vi "SerialTest.vi"() -> ()   [LabVIEW 2014]
doc: "This example performs a serial port write and a serial port read. The parameters set for the serial port must match the parameters of the connected instrument or device. The VISA Configure Serial Port VI sets the configuration parameters. The front panel displays the controls used to configure the basic parameters, such as baud rate, data bits, and parity. The VI passes the VISA resource name to other VIs that perform operations on that VISA resource. The VISA Write function sends a command to the serial device and the VISA Read function returns data based on the command. The VISA Close function then closes the reference to the serial device. It is important to close the reference; otherwise, further communication through that port might not be possible."
uses:
  <vilib>/Instr/_visa.llb/VISA Configure Serial Port (Instr).vi
panel:
  in  "Voltage":dbl min=0.0 max=5000.0 step=0.1 format="%.1f"
  in  "Module":i32=1 min=0 max=5 step=1
  in  "Command":T1(ring)
  out "Response 2":string
  out "Message":string
  in  "Send":bool
  in  "stop":bool
  in  "Command":string="\u000214V1=3244.0v\n"
  out "bytes read":u32
  in  "delay  (ms)":u32=200
  out "Response":string
  in  "VISA resource name":refnum<visa-resource-name>="COM8"
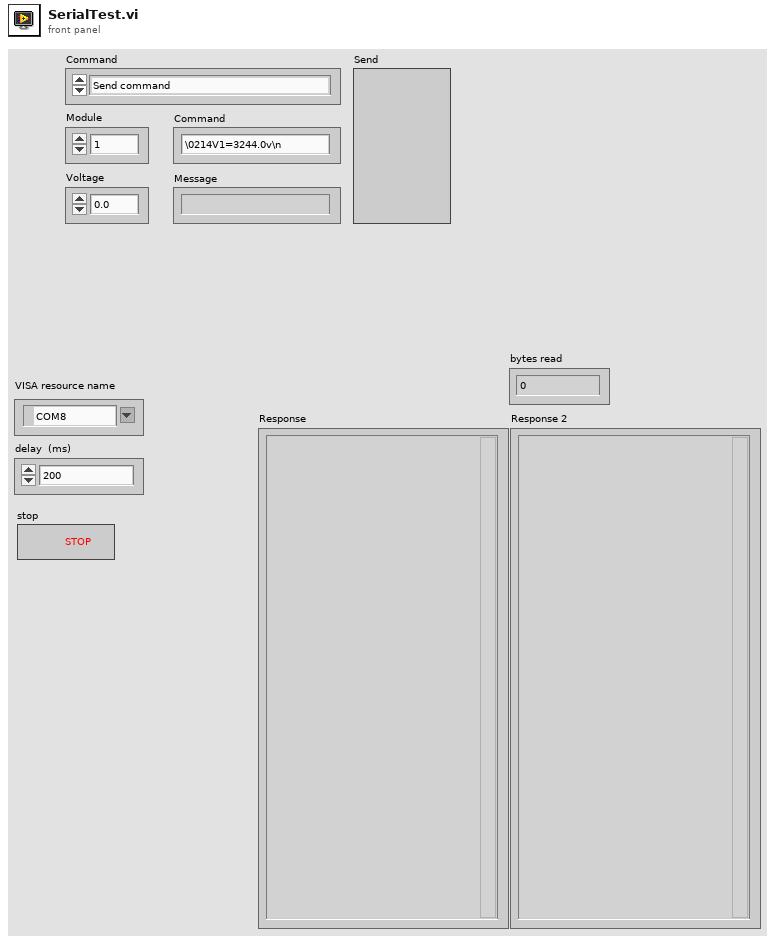
[diagram p1: front panel]
types:
  T1 = enum16{"Send command", "Reset arduino", "Get all set voltages", "Get all actual voltages", "Get all currents", "Get set voltage", "Get actual voltage", "Get current", "Set voltage"}
  T2 = cluster{"baud rate":u32, "data bits":u16, "parity":enum16{"None", "Odd", "Even", "Mark", "Space"}, "stop bits":u16, "flow control":u16}
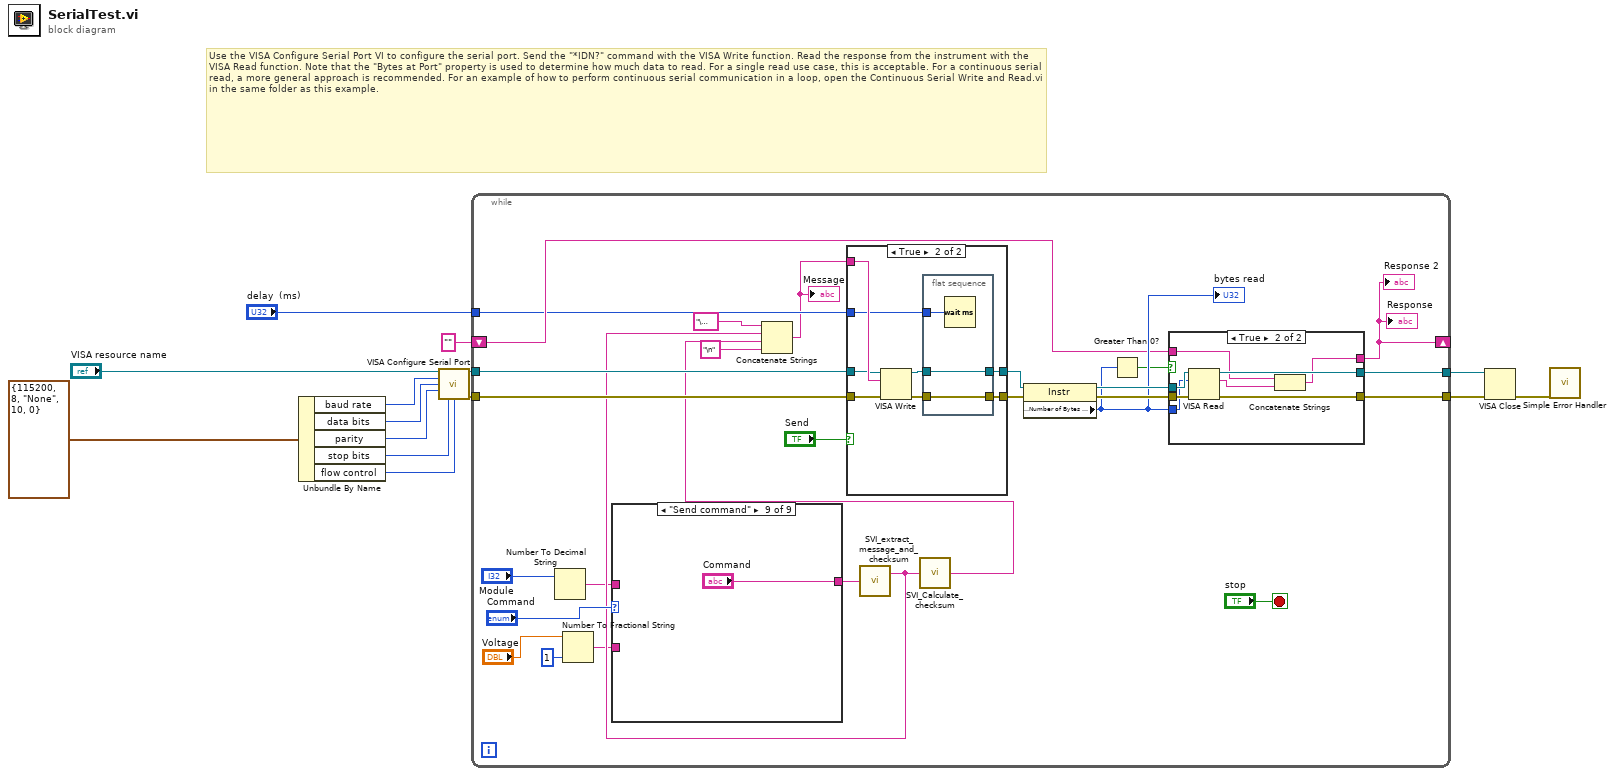
[diagram p0: block diagram]
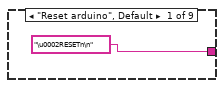
[diagram p2: hidden frame]
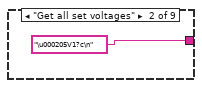
[diagram p3: hidden frame]
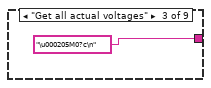
[diagram p4: hidden frame]
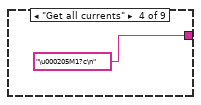
[diagram p5: hidden frame]
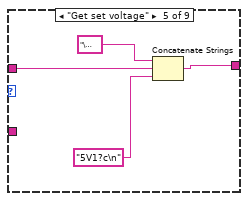
[diagram p6: hidden frame]
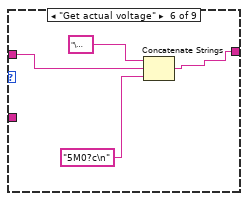
[diagram p7: hidden frame]
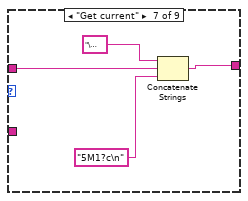
[diagram p8: hidden frame]
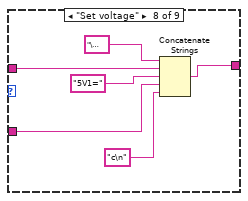
[diagram p9: hidden frame]
diagram:
  # "Use the VISA Configure Serial Port VI to configure the serial port. Send the \"*IDN?\" command with the VISA Write function. Read the response from the instrument with the VISA Read function. Note that the \"Bytes at Port\" property is used to determine how much data to read. For a single read use case, this is acceptable. For a continuous serial read, a more general approach is recommended. For an example of how to perform continuous serial communication in a loop, open the Continuous Serial Write and Read.vi in the same folder as this example."
  n1 = Unbundle By Name(T2 {"baud rate"=115200, "data bits"=8, "parity"=enum."None", "stop bits"=10, "flow control"=0} ("Serial Settings")) -> ("baud rate"=w9:u32, "data bits"=w8:u16, "parity"=w7:enum16{"None", "Odd", "Even", "Mark", "Space"}, "stop bits"=w6:u16, "flow control"=w5:u16)
  n2 = call-poly "VISA Configure Serial Port"("VISA resource name"="VISA resource name", "baud rate (9600)"=w9, "data bits (8)"=w8, "parity (0:none)"=w7, "stop bits (10: 1 bit)"=w6, "flow control (0:none)"=w5) -> ("VISA resource name out"=w4:refnum<visa-resource-name>, "error out"=w2:errorcluster)  [unwired: 3 in, 5 out]
  n3 = while {
    tunnel: [w41] -> w13
    tunnel: [w40] -> w12
    tunnel: w4 -> [w29]
    tunnel: "delay  (ms)" -> [w30]
    tunnel: w2 -> [w28]
    shift-right: [w24] -> _
    shift-left: "" ("read buffer") -> [w31]
    stop <- "stop" stop-if-true
    n4 = Number To Decimal String(number="Module") -> (decimal integer string=w18:string)  [unwired: 1 in]
    n5 = Number To Fractional String(number="Voltage", precision (6)=i16 1) -> (F-format string=w16:string)  [unwired: 2 in]
    n6 = case shown="\"Send command\"" "Command" {
      tunnel: ["\u0002RESETn\n" ("string") "\u000205V1?c\n" ("string") "\u000205M0?c\n" ("string") "\u000205M1?c\n" ("string") w47 w52 w56 w62 "Command"] -> w22
      tunnel: w18 -> [_ _ _ _ w48 w51 w55 w61 _]
      tunnel: w16 -> [_ _ _ _ _ _ _ w59 _]
      frame "Reset arduino", Default {
      }
      frame "Get all set voltages" {
      }
      frame "Get all actual voltages" {
      }
      frame "Get all currents" {
      }
      frame "Get set voltage" {
        n7 = Concatenate Strings("\u0002" ("string"), w48, "5V1?c\n" ("string")) -> (w47:string)
      }
      frame "Get actual voltage" {
        n8 = Concatenate Strings("\u0002" ("string"), w51, "5M0?c\n" ("string")) -> (w52:string)
      }
      frame "Get current" {
        n9 = Concatenate Strings("\u0002" ("string"), w55, "5M1?c\n" ("string")) -> (w56:string)
      }
      frame "Set voltage" {
        n10 = Concatenate Strings("\u0002" ("string"), w61, "5V1=" ("string"), w59, "c\n" ("string")) -> (w62:string)
      }
      frame "Send command" {
      }
    }
    n11 = call "SVI_extract_message_and_checksum.vi"("String in"=w22) -> ("Message"=w21:string)  [unwired: 1 out]
    n12 = call "SVI_Calculate_checksum.vi"("Message"=w21) -> ("Calculated checksum"=w20:string)
    n13 = Concatenate Strings("\u0002" ("string"), w21, w20, "\n" ("string")) -> (w27:string)
    "Message" <- w27
    n14 = case shown="True" "Send" {
      tunnel: [w77 w84] -> w39
      tunnel: [w76 w82] -> w38
      tunnel: w27 -> [_ w81]
      tunnel: w30 -> [_ w80]
      tunnel: w28 -> [w77 w79]
      tunnel: w29 -> [w76 w78]
      frame False {
      }
      frame True {
        n15 = VISA Write(VISA resource name=w78, write buffer=w81, error in (no error)=w79) -> (VISA resource name out=w83:refnum<visa-resource-name>, error out=w85:errorcluster)  [unwired: 1 out]
        n16 = flat-sequence {
          tunnel: w85 -> [w87]
          tunnel: [w87] -> w84
          tunnel: w83 -> [w86]
          tunnel: [w86] -> w82
          tunnel: w80 -> [w88]
          frame #0 {
            n17 = Wait (ms)(milliseconds to wait=w88) -> ()  [unwired: 1 out]
          }
        }
      }
    }
    n18 = property class="Instr"(reference=w38, error in=w39) -> (reference out=w37:refnum<visa-resource-name>, error out=w36:errorcluster, "Serial Settings:Number of Bytes at Serial Port"=w33:u32)
    "bytes read" <- w33
    n19 = Greater Than 0?(x=w33) -> (x > 0?=w32:bool)
    n20 = case shown="True" w32 {
      tunnel: [w66 w75] -> w41
      tunnel: [w65 w74] -> w40
      tunnel: w37 -> [w65 w73]
      tunnel: w36 -> [w66 w72]
      tunnel: [w67 w68] -> w24
      tunnel: w33 -> [_ w71]
      tunnel: w31 -> [w67 w70]
      frame False {
      }
      frame True {
        n21 = VISA Read(VISA resource name=w73, byte count=w71, error in (no error)=w72) -> (VISA resource name out=w74:refnum<visa-resource-name>, read buffer=w69:string, error out=w75:errorcluster)  [unwired: 1 out]
        n22 = Concatenate Strings(w70, w69) -> (w68:string)
      }
    }
    "Response" <- w24
    "Response 2" <- w24
  }
  n23 = VISA Close(VISA resource name=w12, error in (no error)=w13) -> (error out=w11:errorcluster)
  n24 = call <vilib>:"Simple Error Handler.vi"("error in (no error)"=w11) -> ()  [unwired: 1 in, 8 out]
